vi "GetName.vi"(8 "error in (no error)":errorcluster, 11 "TestSuite in":refnum<class "TestSuite.lvclass">) -> (0 "error out":errorcluster, 2 "Name":string, 3 "TestSuite out":refnum<class "TestSuite.lvclass">)   [LabVIEW 2019, in "TestSuite.lvclass"]
doc: "Returns the name."
uses:
  TestSuite.lvclass
  TestSuite.lvclass/TestSuite.ctl
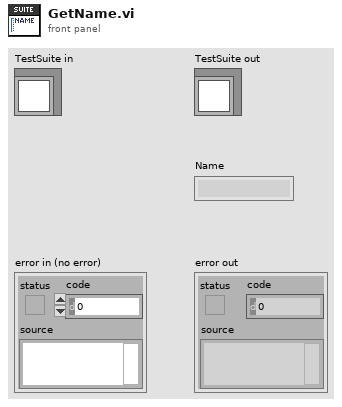
[diagram p1: front panel]
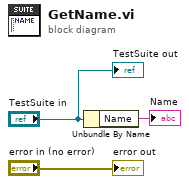
[diagram p0: block diagram]
diagram:
  n1 = Unbundle By Name("TestSuite in") -> ("Name"=→"Name":string)
  "error out" <- "error in (no error)"
  "TestSuite out" <- "TestSuite in"
